vi "data_output_continuous.vi"() -> ()   [LabVIEW 2016]
uses:
  <vilib>/Utility/error.llb/DialogType.ctl
  <vilib>/DAQmx/configure/timing.llb/DAQmx Timing (Sample Clock).vi
  <resource>/objmgr/daqmx.rc
  <vilib>/DAQmx/write.llb/DAQmx Write (Analog 1D Wfm NChan NSamp).vi
  <vilib>/DAQmx/read.llb/DAQmx Read (Digital Wfm 1Chan NSamp).vi
  <vilib>/Waveform/DTblOps.llb/DTbl Digital to Boolean Array.vi
  <vilib>/DAQmx/create/channels.llb/DAQmx Create Channel (DI-Digital Input).vi
  <vilib>/DAQmx/create/channels.llb/DAQmx Create Channel (AO-Voltage-Basic).vi
  <vilib>/Analysis/Matrix/NI_Matrix.lvlib
  <vilib>/Analysis/Matrix/Numeric/Add/Add (Elementwise) - R,RM.vi
  <vilib>/Utility/file.llb/Read Delimited Spreadsheet (DBL).vi
panel:
  out "Multiplier 3":dbl
  out "Multiplier 2":dbl
  out "Ventricle Squash":bool
  out "Atrial Squash":bool
  out "Signal Squash":bool
  in  "Samples per Loop":i32=1000
  out "Digital Waveform Graph":digitalwaveform(graph)
  in  "Sample Rate 2":dbl=1000.0
  in  "Sample Clock Source 2":tag="PFI0"
  out "Actual Sample Rate":dbl=1000.0 format="%0.2f"
  in  "Digital Input Lines":tag="Dev1/port0/line0:7"
  out "Waveform Graph 2":dynamicdata(graph)
  out "Multiplier":dbl
  in  "Sample Rate":dbl=1000.0
  in  "Sample Clock Source":tag="OnboardClock"
  in  "Max Voltage":dbl=5.0
  in  "Min Voltage":dbl=-5.0
  in  "Analog Output Physical Channel(s)":tag="Dev1/ao0"
  in  "Stop":bool
  out "Number of Samples Written per Channel":dbl
  out "Waveform Graph":dynamicdata(graph)
  out "Matrix Cols":dbl
  out "Matrix Rows":dbl
  in  "csv Path":path
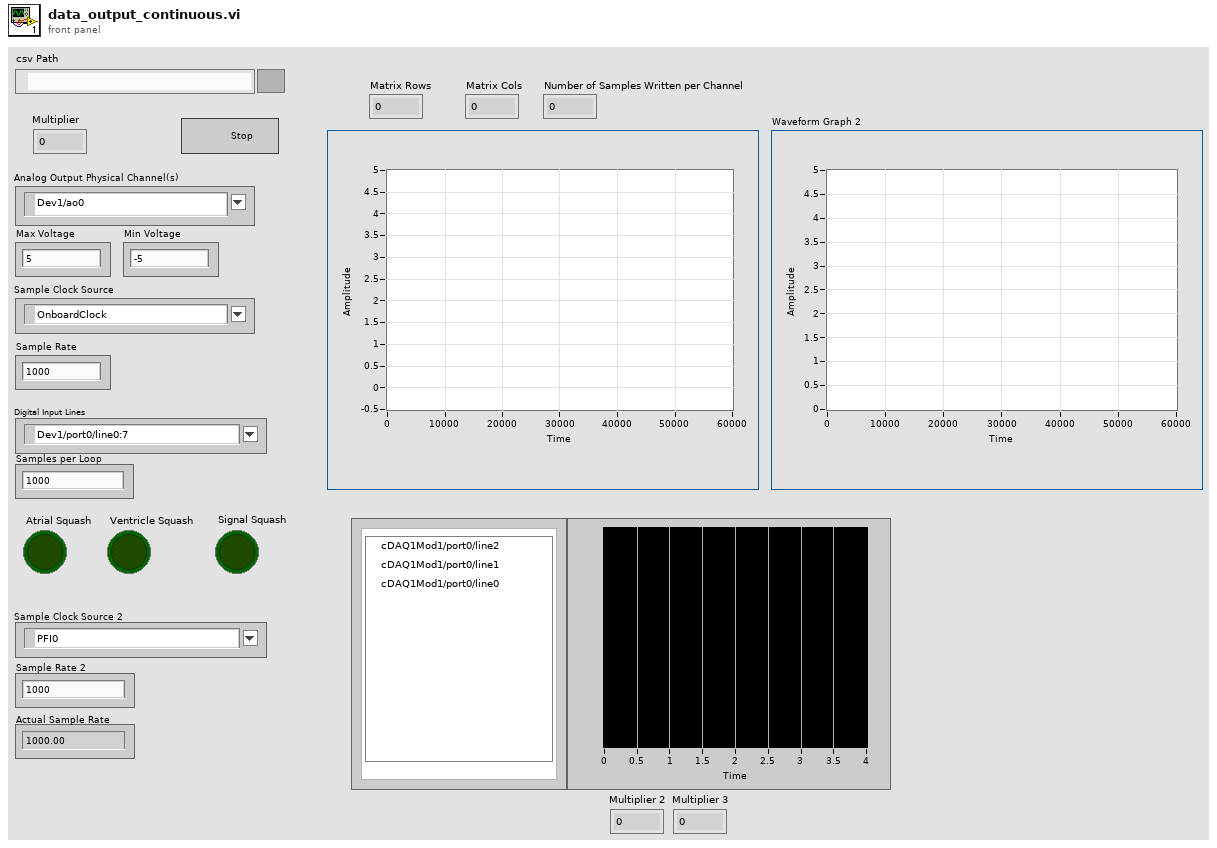
[diagram p1: front panel]
types:
  T1 = typedef "DialogType.ctl" = u16
  T2 = typedef "NI_Matrix.lvlib/RealMatrix.ctl" = dbl[][]
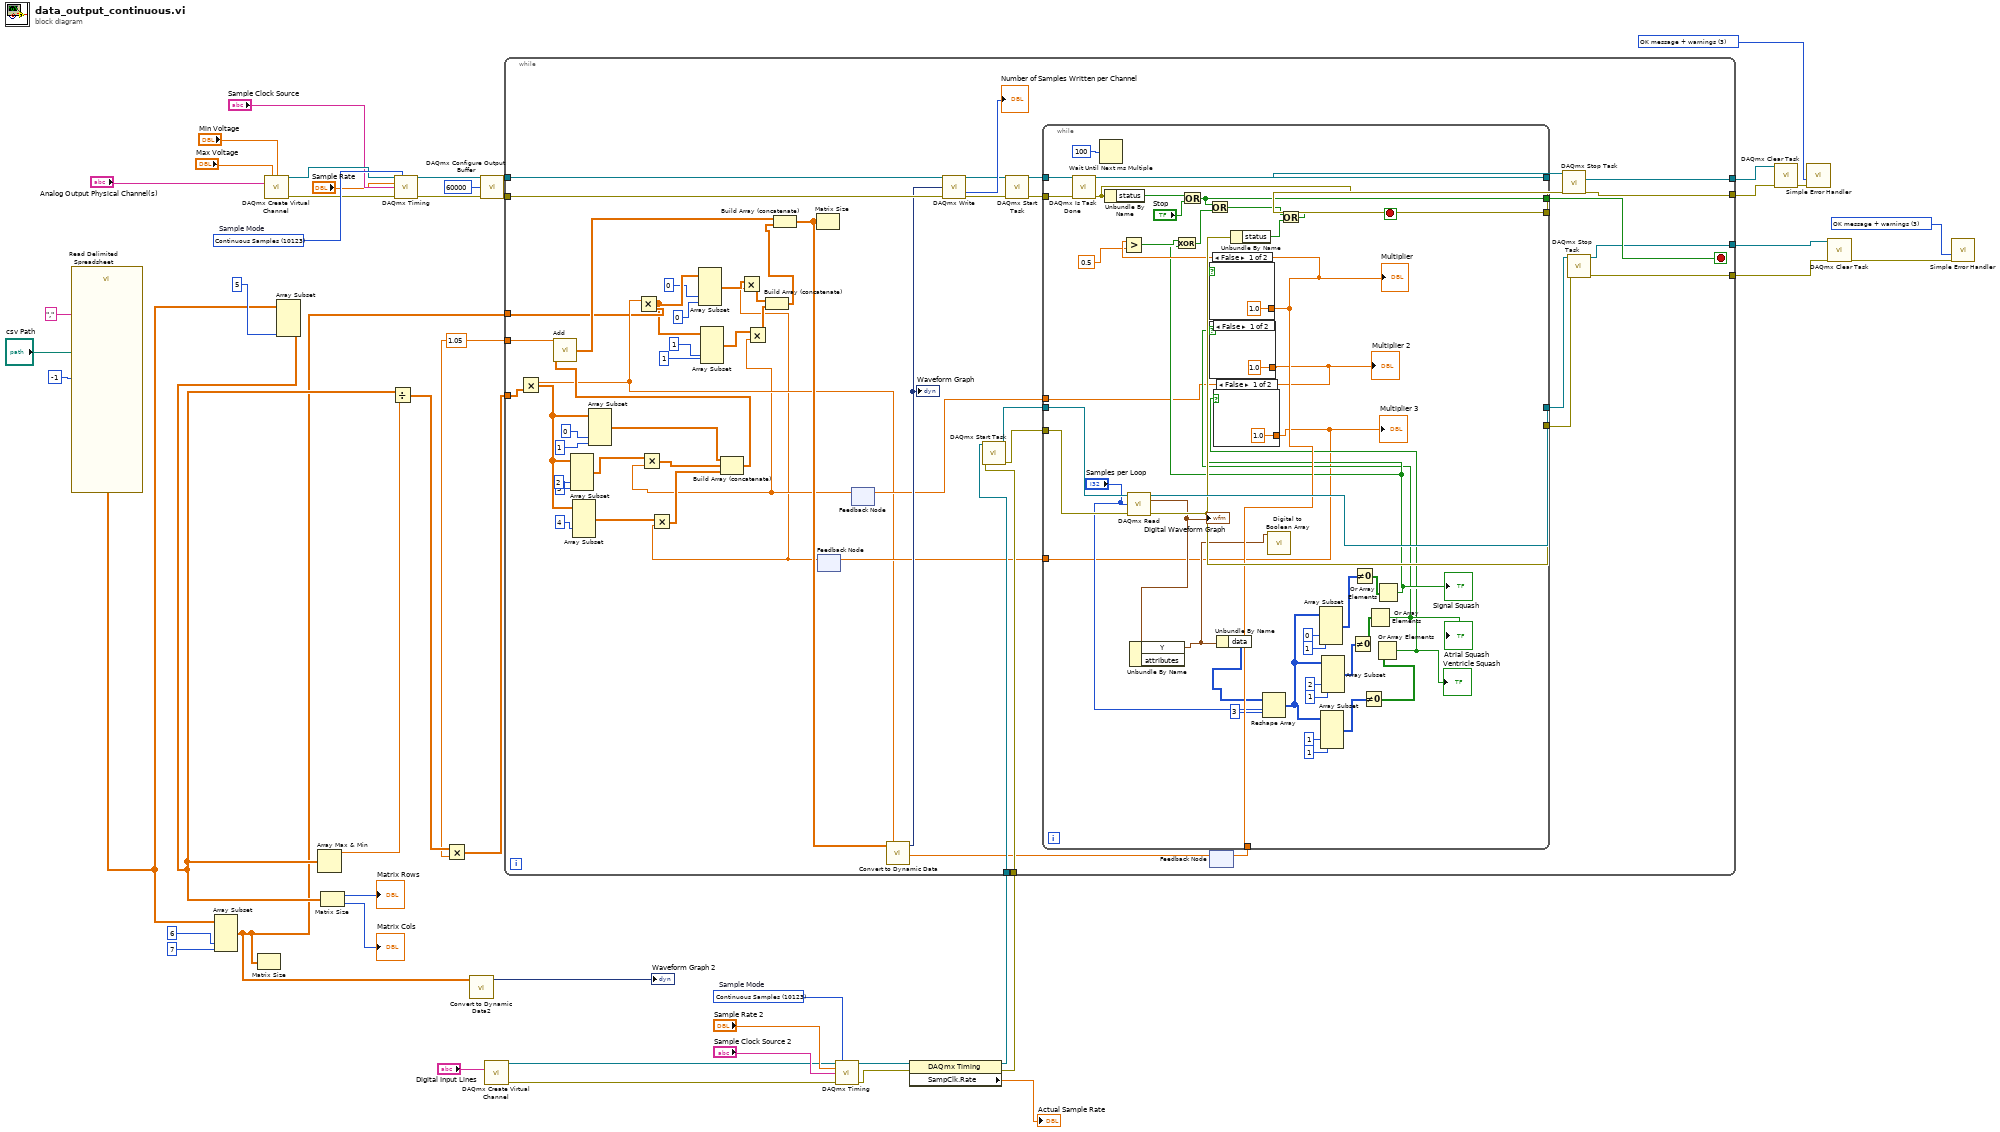
[diagram p0: block diagram]
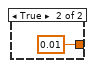
[diagram p2: hidden frame]
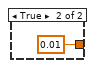
[diagram p3: hidden frame]
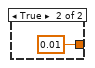
[diagram p4: hidden frame]
diagram:
  w6 = T1 3 items=["no dialog", "OK message", "continue or stop message", "OK message + warnings", "continue/stop + warnings"] ("type of dialog (OK msg:1)")
  w15 = 10123 items=["Finite Samples"=10178, "Continuous Samples"=10123, "Hardware Timed Single Point"=12522]  # Sample Mode
  w39 = 10123 items=["Finite Samples"=10178, "Continuous Samples"=10123, "Hardware Timed Single Point"=12522]  # Sample Mode
  w40 = T1 3 items=["no dialog", "OK message", "continue or stop message", "OK message + warnings", "continue/stop + warnings"] ("type of dialog (OK msg:1)")
  w17 = 1.05
  n1 = call-poly <vilib>:"Read Delimited Spreadsheet.vi"("file path (dialog if empty)"="csv Path", "number of rows (all:-1)"=-1, "delimiter (\\t)"=",") -> ("all rows"=w22:dbl[][])  [unwired: 7 in, 5 out]
  n2 = Array Subset(array=w22, index (col)=6, length (col)=7) -> (w18:dbl[][])  [unwired: 2 in]
  n3 = Matrix Size(0:w18) -> ()  [unwired: 2 out]
  n4 = call-poly <vilib>:"DAQmx Create Virtual Channel.vi"("maximum value"="Max Voltage", "minimum value"="Min Voltage", "physical channels"="Analog Output Physical Channel(s)") -> ("task out"=w37:refnum<k21>, "error out"=w38:errorcluster)  [unwired: 11 in]
  n5 = Array Subset(array=w22, length (col)=5) -> (w24:dbl[][])  [unwired: 3 in]
  n6 = Array Max & Min(array=w24) -> (max value=w45:dbl)  [unwired: 3 out]
  n7 = Matrix Size(0:w24) -> (1:→"Matrix Rows":i32, 2:→"Matrix Cols":i32)
  n8 = Divide(x=w24, y=w45) -> (x/y=w44:dbl[][])
  n9 = call-poly <vilib>:"DAQmx Timing.vi"("task/channels in"=w37, "sample mode"=w39, "rate"="Sample Rate", "source"="Sample Clock Source", "error in"=w38) -> ("task out"=w31:refnum<k21>, "error out"=w29:errorcluster)  [unwired: 9 in]
  n10 = Multiply(x=w44, y=w17) -> (x*y=w1:dbl[][])
  n11 = call "Convert to Dynamic Data2"("2D Array"=w18) -> ("Dynamic Data Type"=→"Waveform Graph 2":dynamicdata)  [unwired: 3 in]
  n12 = call <vilib>:"DAQmx Configure Output Buffer.vi"("task/channels in"=w31, "buffer size (in samples per channel)"=60000, "error in"=w29) -> ("task out"=w28:refnum<k21>, "error out"=w27:errorcluster)  [unwired: 11 in]
  n13 = call-poly <vilib>:"DAQmx Create Virtual Channel.vi"("lines"="Digital Input Lines") -> ("task out"=w12:refnum<k21>, "error out"=w11:errorcluster)  [unwired: 13 in]
  n14 = call-poly <vilib>:"DAQmx Timing.vi"("task/channels in"=w12, "sample mode"=w15, "rate"="Sample Rate 2", "source"="Sample Clock Source 2", "error in"=w11) -> ("task out"=w10:refnum<k21>, "error out"=w9:errorcluster)  [unwired: 9 in]
  n15 = property class="DAQmx Timing"(reference=w10, error in=w9) -> (reference out=w3:refnum<k21>, error out=w2:errorcluster, "SampClk.Rate"=→"Actual Sample Rate":dbl)
  n16 = while {
    tunnel: w28 -> [w97]
    tunnel: w27 -> [w96]
    tunnel: w1 -> [w93]
    tunnel: [w90] -> w26
    tunnel: [w89] -> w25
    tunnel: w18 -> [w61]
    tunnel: w17 -> [w86]
    tunnel: [w84] -> w5
    tunnel: [w83] -> w4
    tunnel: w3 -> [w80]
    tunnel: w2 -> [w79]
    stop <- w94 stop-if-true
    n17 = feedback #1() -> (w49:dbl)  [unwired: 1 in]
    n18 = feedback #2() -> (w50:dbl)  [unwired: 1 in]
    n19 = call <vilib>:"DAQmx Start Task.vi"("task/channels in"=w80, "error in"=w79) -> ("task out"=w77:refnum<k21>, "error out"=w78:errorcluster)  [unwired: 12 in]
    n20 = feedback #3() -> (w62:dbl)  [unwired: 1 in]
    n21 = Multiply(x=w62, y=w93) -> (x*y=w66:dbl[][])
    n22 = Array Subset(array=w66, index (col)=2 ("column 1"), length (col)=3 ("column N")) -> (w70:dbl[][])  [unwired: 2 in]
    n23 = Array Subset(array=w66, index (col)=4 ("column 1")) -> (w69:dbl[][])  [unwired: 3 in]
    n24 = Array Subset(array=w66, index (col)=0 ("column 1"), length (col)=1 ("column N")) -> (w71:dbl[][])  [unwired: 2 in]
    n25 = Multiply(x=w62, y=w61) -> (x*y=w60:dbl[][])
    n26 = Multiply(x=w70, y=w50) -> (x*y=w67:dbl[][])
    n27 = Multiply(x=w69, y=w49) -> (x*y=w68:dbl[][])
    n28 = Array Subset(array=w60, index (col)=0 ("column 1"), length (col)=0 ("column N")) -> (w53:dbl[][])  [unwired: 2 in]
    n29 = Array Subset(array=w60, index (col)=1 ("column 1"), length (col)=1 ("column N")) -> (w54:dbl[][])  [unwired: 2 in]
    n30 = Build Array (concatenate)(w71, w67, w68) -> (w65:T2)
    n31 = call-poly <vilib>:"Add.vi"("Real Matrix A"=w65, "Real Scalar c"=w86) -> ("c + A"=w85:T2)
    n32 = Multiply(x=w53, y=w49) -> (x*y=w52:dbl[][])
    n33 = Multiply(x=w54, y=w50) -> (x*y=w51:dbl[][])
    n34 = Build Array (concatenate)(w52, w51) -> (w59:T2)
    n35 = Build Array (concatenate)(w85, w59) -> (w87:T2)
    n36 = Matrix Size(0:w87) -> ()  [unwired: 2 out]
    n37 = call "Convert to Dynamic Data"("2D Array"=w87) -> ("Dynamic Data Type"=w95:dynamicdata)  [unwired: 3 in]
    "Waveform Graph" <- w95
    n38 = call-poly <vilib>:"DAQmx Write.vi"("task/channels in"=w97, "data"=w95, "error in"=w96) -> ("task out"=w101:refnum<k21>, "number of samples written per channel"=→"Number of Samples Written per Channel":u32, "error out"=w100:errorcluster)  [unwired: 10 in]
    n39 = call <vilib>:"DAQmx Start Task.vi"("task/channels in"=w101, "error in"=w100) -> ("task out"=w98:refnum<k21>, "error out"=w99:errorcluster)  [unwired: 12 in]
    n40 = while {
      tunnel: w98 -> [w141]
      tunnel: w99 -> [w140]
      tunnel: [w139] -> w94
      tunnel: [w138] -> w92
      tunnel: [w137] -> w91
      tunnel: [w129] -> w88
      tunnel: [w136] -> w82
      tunnel: [w135] -> w81
      tunnel: w78 -> [w134]
      tunnel: w77 -> [w133]
      tunnel: [w104] -> w64
      tunnel: [w103] -> w63
      stop <- w130 stop-if-true
      n41 = call <vilib>:"DAQmx Is Task Done.vi"("task/channels in"=w141, "error in"=w140) -> ("task out"=w138:refnum<k21>, "error out"=w137:errorcluster)  [unwired: 11 in, 1 out]
      n42 = Wait Until Next ms Multiple(millisecond multiple=u32 100) -> ()  [unwired: 1 out]
      n43 = Unbundle By Name(w137) -> ("status"=w144:bool)
      n44 = call-poly <vilib>:"DAQmx Read.vi"("task/channels in"=w133, "number of samples per channel"="Samples per Loop", "error in"=w134) -> ("task out"=w136:refnum<k21>, "data"=w124:digitalwaveform, "error out"=w135:errorcluster)  [unwired: 10 in]
      "Digital Waveform Graph" <- w124
      n45 = Unbundle By Name(w124) -> ("Y"=w121:digitaldata)  [unwired: 1 out]
      n46 = Or(x=w144, y="Stop") -> (x .or. y?=w139:bool)
      n47 = Unbundle By Name(w121) -> ("data"=w107:u8[][])
      n48 = Unbundle By Name(w135) -> ("status"=w131:bool)
      n49 = Reshape Array(w107, "Samples per Loop", 3 ("dimension size")) -> (w105:u8[][])
      n50 = call-poly <vilib>:"Digital to Boolean Array.vi"("digital data"=w121) -> ()  [unwired: 9 in, 2 out]
      n51 = Array Subset(array=w105, index (col)=0 ("index"), length (col)=1 ("length")) -> (w114:u8[][])  [unwired: 2 in]
      n52 = Array Subset(array=w105, index (col)=1 ("index"), length (col)=1 ("length")) -> (w106:u8[][])  [unwired: 2 in]
      n53 = Array Subset(array=w105, index (col)=2 ("index"), length (col)=1 ("length")) -> (w108:u8[][])  [unwired: 2 in]
      n54 = Not Equal To 0?(x=w108) -> (x != 0?=w123:bool[][])
      n55 = Not Equal To 0?(x=w114) -> (x != 0?=w113:bool[][])
      n56 = Not Equal To 0?(x=w106) -> (x != 0?=w122:bool[][])
      n57 = Or Array Elements(Boolean array=w123) -> (logical OR=w118:bool)
      "Atrial Squash" <- w118
      n58 = case shown="False" w118 {
        tunnel: [1.0 0.01] -> w104
        frame False {
        }
        frame True {
        }
      }
      "Multiplier 2" <- w104
      n59 = Or Array Elements(Boolean array=w122) -> (logical OR=w117:bool)
      "Ventricle Squash" <- w117
      n60 = case shown="False" w117 {
        tunnel: [1.0 0.01] -> w103
        frame False {
        }
        frame True {
        }
      }
      "Multiplier 3" <- w103
      n61 = Or Array Elements(Boolean array=w113) -> (logical OR=w126:bool)
      "Signal Squash" <- w126
      n62 = case shown="False" w126 {
        tunnel: [1.0 0.01] -> w129
        frame False {
        }
        frame True {
        }
      }
      "Multiplier" <- w129
      n63 = Greater?(x=w129, y=0.5) -> (0:w127:bool)
      n64 = Exclusive Or(1:w126, 2:w127) -> (0:w125:bool)
      n65 = Or(x=w139, y=w125) -> (x .or. y?=w132:bool)
      n66 = Or(x=w132, y=w131) -> (x .or. y?=w130:bool)
    }
    n67 = feedback-in #1(w63) -> ()
    n68 = feedback-in #2(w64) -> ()
    n69 = feedback-in #3(w88) -> ()
    n70 = call <vilib>:"DAQmx Stop Task.vi"("task/channels in"=w92, "error in"=w91) -> ("task out"=w90:refnum<k21>, "error out"=w89:errorcluster)  [unwired: 12 in]
    n71 = call <vilib>:"DAQmx Stop Task.vi"("task/channels in"=w82, "error in"=w81) -> ("task out"=w84:refnum<k21>, "error out"=w83:errorcluster)  [unwired: 12 in]
  }
  n72 = call <vilib>:"DAQmx Clear Task.vi"("task in"=w26, "error in"=w25) -> ("error out"=w41:errorcluster)  [unwired: 13 in]
  n73 = call <vilib>:"Simple Error Handler.vi"("type of dialog (OK msg:1)"=w40, "error in (no error)"=w41) -> ()  [unwired: 3 in, 5 out]
  n74 = call <vilib>:"DAQmx Clear Task.vi"("task in"=w5, "error in"=w4) -> ("error out"=w7:errorcluster)  [unwired: 13 in]
  n75 = call <vilib>:"Simple Error Handler.vi"("type of dialog (OK msg:1)"=w6, "error in (no error)"=w7) -> ()  [unwired: 3 in, 5 out]
